vi "Generate Trace.vi"(10 "Trace String":string, 11 "AF Trace Format in":refnum<class "AF Trace Format.lvclass">) -> (3 "AF Trace Format out":refnum<class "AF Trace Format.lvclass">)   [LabVIEW 2020, in "Actor Framework.lvlib" / "AF Trace Format.lvclass"]
uses:
  AF Trace Format.lvclass
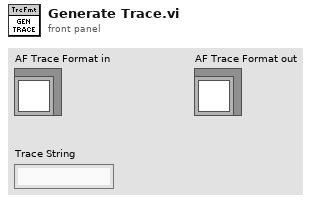
[diagram p1: front panel]
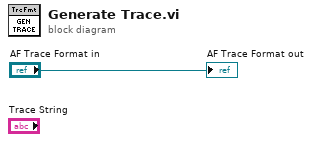
[diagram p0: block diagram]
diagram:
  "AF Trace Format out" <- "AF Trace Format in"
